vi "BRig_arrTrig_L_Selection_event_l1.vi"() -> (2 "output_L_Sel_event_l1":i32)   [LabVIEW 2014]
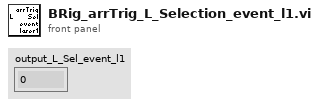
[diagram p1: front panel]
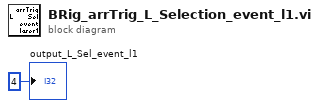
[diagram p0: block diagram]
diagram:
  "output_L_Sel_event_l1" <- 4
